vi "Read Time (ms).vi"(8 "error in (no error)":errorcluster, 11 "Wait in":refnum<class "Wait.lvclass">) -> (0 "error out":errorcluster, 2 "Time (ms)":u32, 3 "Wait out":refnum<class "Wait.lvclass">)   [LabVIEW 2021, in "BT.lvlib" / "Wait.lvclass"]
uses:
  Wait.lvclass
  Wait.lvclass/Wait.ctl
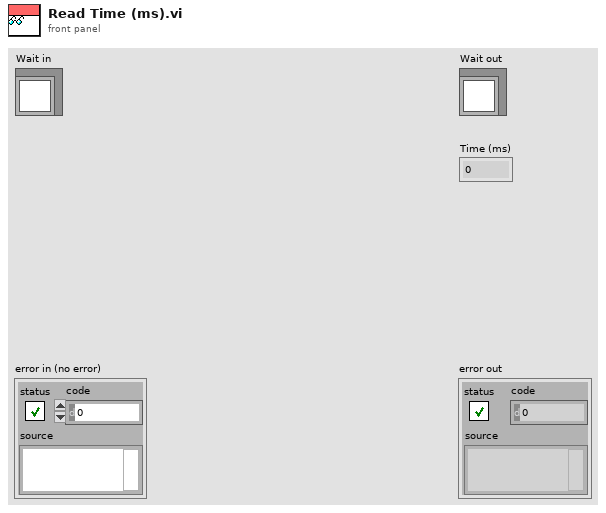
[diagram p1: front panel]
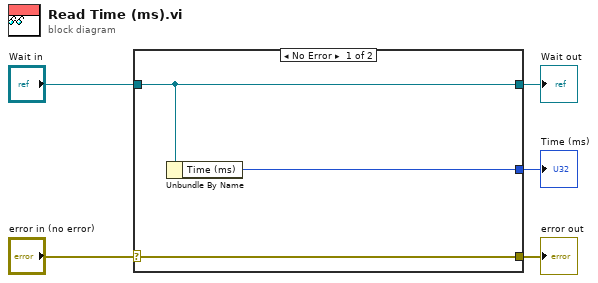
[diagram p0: block diagram]
diagram:
  n1 = case shown="No Error" "error in (no error)" {
    selector: "error in (no error)" -> [w8 w9]
    tunnel: [w8 w9] -> w4
    tunnel: [w7 w10] -> w2
    tunnel: "Wait in" -> [w7 w10]
    tunnel: [w6 _] -> w1
    frame No Error {
      n2 = Unbundle By Name(w7) -> ("Time (ms)"=w6:u32)
    }
    frame Error {
    }
  }
  "error out" <- w4
  "Wait out" <- w2
  "Time (ms)" <- w1
